vi "MCS_CloseSystem.vi"(1 "error in (no error)":errorcluster, 2 "System Index In":u32) -> (0 "error out":errorcluster)   [LabVIEW 2010]
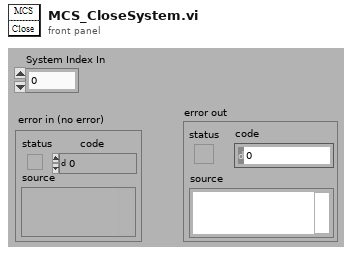
[diagram p1: front panel]
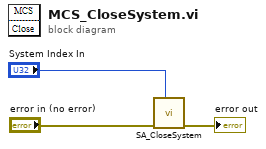
[diagram p0: block diagram]
diagram:
  n1 = call <vilib>:"SA_CloseSystem.vi"("systemIndex"="System Index In", "error in (no error)"="error in (no error)") -> ("error out"=→"error out":errorcluster)  [unwired: 9 in]
